vi "GetValue.vi"(8 "error in (no error)":errorcluster, 10 "Key":variant, 11 "Map in":refnum<class "Map.lvclass">) -> (0 "error out":errorcluster, 1 "Invalid?":bool, 2 "Value":variant, 3 "Map out":refnum<class "Map.lvclass">)   [LabVIEW 2016, in "Map.lvclass"]
uses:
  <userlib>/836-libraries/Data_Structures/Map/Map.lvclass
  <userlib>/836-libraries/Data_Structures/Map/Map.lvclass/Map.ctl
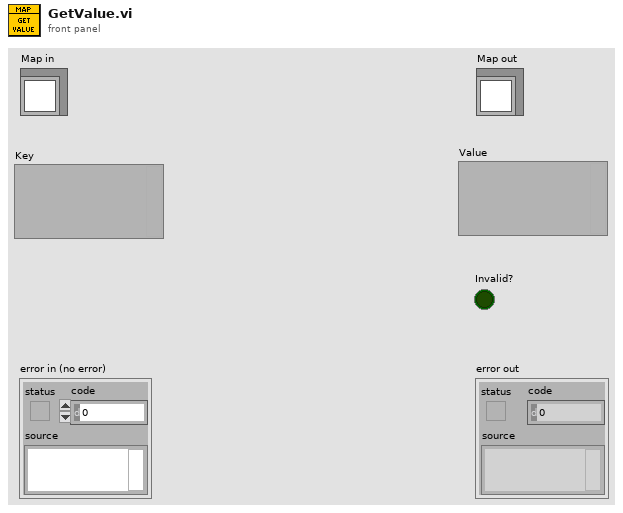
[diagram p1: front panel]
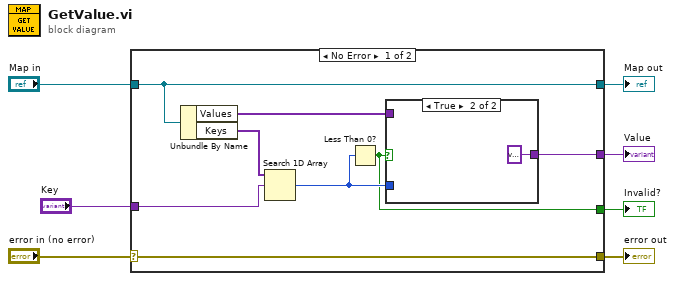
[diagram p0: block diagram]
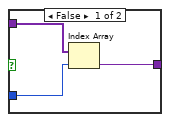
[diagram p2: hidden frame]
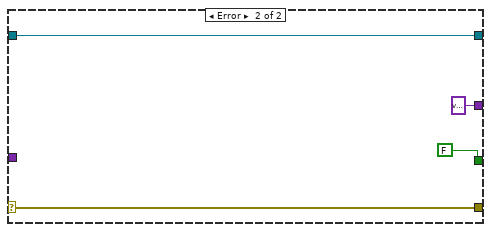
[diagram p3: hidden frame]
diagram:
  n1 = case shown="No Error" "error in (no error)" {
    selector: "error in (no error)" -> [w15 w22]
    tunnel: [w15 w22] -> w6
    tunnel: [w14 w23] -> w4
    tunnel: "Map in" -> [w14 w23]
    tunnel: "Key" -> [w12 _]
    tunnel: [w9 variant ("Key")] -> w2
    tunnel: [w8 FALSE] -> w1
    frame No Error {
      n2 = Unbundle By Name(w14) -> ("Values"=w11:variant[], "Keys"=w13:variant[])
      n3 = Search 1D Array(1D array=w13, element=w12) -> (index of element=w10:i32)  [unwired: 1 in]
      n4 = Less Than 0?(x=w10) -> (x < 0?=w8:bool)
      n5 = case shown="True" w8 {
        tunnel: w11 -> [w18 _]
        tunnel: w10 -> [w17 _]
        tunnel: [w16 variant ("Key")] -> w9
        frame False {
          n6 = Index Array(array=w18, index=w17) -> (element=w16:variant)
        }
        frame True {
        }
      }
    }
    frame Error {
    }
  }
  "error out" <- w6
  "Map out" <- w4
  "Value" <- w2
  "Invalid?" <- w1
